vi "Main.vi"() -> ()   [LabVIEW 2020]
panel:
  out "Tab Control":enum32{"Page 1", "Page 2", "Page 3"}(tab)
  in  "Abort Button":bool
  in  "Tabs buttons":enum32{"Button 1", "Button 2", "Button 3"}(radio)
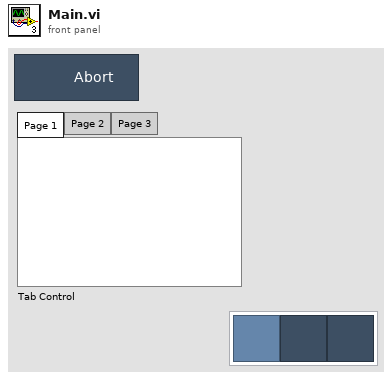
[diagram p1: front panel]
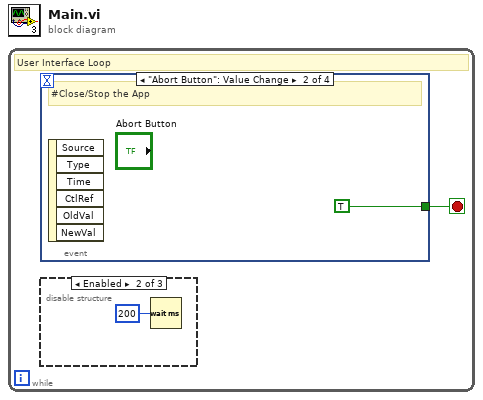
[diagram p0: block diagram]
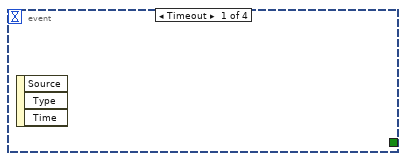
[diagram p2: hidden frame]
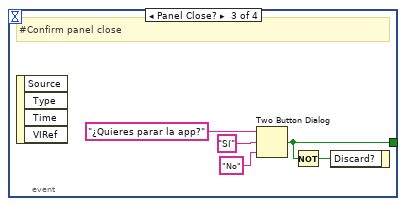
[diagram p3: hidden frame]
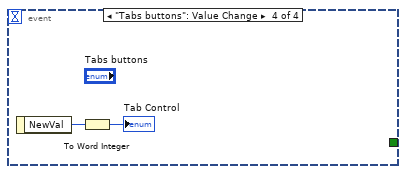
[diagram p4: hidden frame]
diagram:
  n1 = while {
    stop <- w1 stop-if-true
    # "User Interface Loop"
    n2 = event shown="[1] \"Abort Button\": Value Change" {
      selector: _ -> [_ _ _ _]
      dyn-events: _ -> [_ _ _ _]
      timeout: _ -> [_ _ _ _]
      tunnel: [_ TRUE ("Abort Button") w3 _] -> w1
      event Timeout {
        n3 = event-data() -> ()  [unwired: 1 in, 3 out]
      }
      event "Abort Button": Value Change {
        # "#Close/Stop the App"
        n4 = event-data() -> ()  [unwired: 1 in, 6 out]
      }
      event Panel Close? {
        # "#Confirm panel close"
        n5 = event-data() -> ()  [unwired: 1 in, 4 out]
        n6 = Two Button Dialog(message="¿Quieres parar la app?", 1:"No" ("F button name (\"Cancel\")"), 2:"Sí" ("T button name (\"OK\")")) -> (T button?=w3:bool)
        n7 = Not(x=w3) -> (.not. x?=w4:bool)
        n8 = event-data("Discard?"=w4) -> ()  [unwired: 1 in, 1 out]
      }
      event "Tabs buttons": Value Change {
        n9 = event-data() -> ("NewVal"=w9:enum32{"Button 1", "Button 2", "Button 3"})  [unwired: 1 in]
        n10 = To Word Integer(number=w9) -> (16bit integer=→"Tab Control":i16)
      }
    }
    n11 = disable-structure shown="Enabled" {
      frame Disabled {
      }
      frame Enabled {
        n12 = Wait (ms)(milliseconds to wait=u32 200 ("millisecond multiple")) -> ()  [unwired: 1 out]
      }
      frame Disabled {
      }
    }
  }
